vi "XY Graph Set Selected Plots.vi"(8 "Error In":errorcluster, 9 "Selected Plots":i32[](array[numeric]), 11 "XY Graph Refnum":T1) -> (0 "Error Out":errorcluster, 1 "Selected Plot Names":string[](array[string]), 2 "Caption (or Label) Text":string, 3 "XY Graph Refnum (dup)":T1)   [LabVIEW 2021, in "XY Graph Add-Ons.lvlib"]
uses:
  XY Graph Refnum.ctl
  XY Graph Add-Ons.lvlib
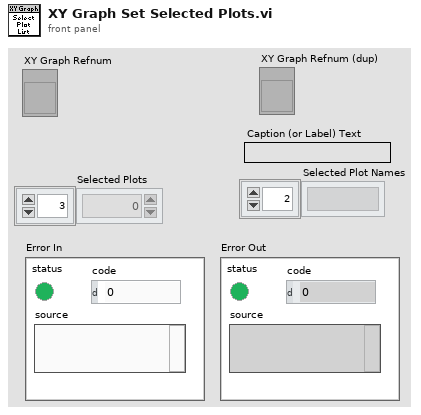
[diagram p1: front panel]
types:
  T1 = typedef "XY Graph Add-Ons.lvlib/XY Graph Refnum.ctl" = refnum<vi>
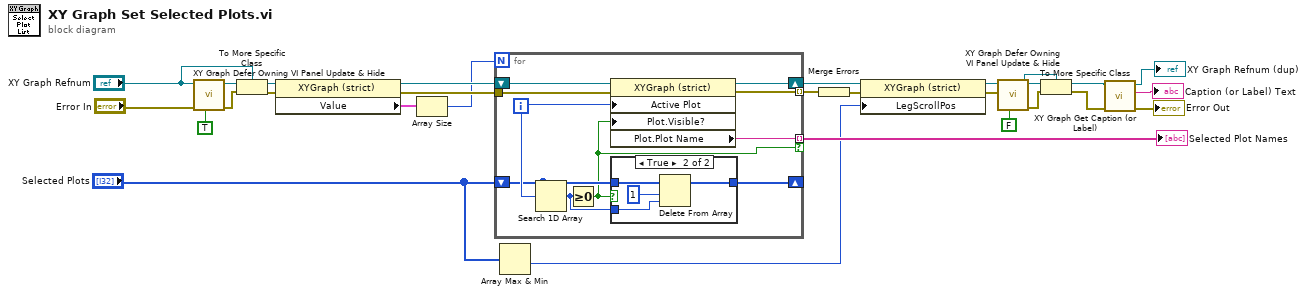
[diagram p0: block diagram]
diagram:
  n1 = call "XY Graph Defer Owning VI Panel Update & Hide.vi"("Defer Owning Panel Update"=TRUE ("Hide (F)/Show (T) Graph"), "error in (no error)"="Error In", "XY Graph Refnum in"="XY Graph Refnum") -> ("error out"=w19:errorcluster, "XY Graph Refnum out"=w21:refnum<vi>)  [unwired: 7 in]
  n2 = To More Specific Class(target class="XY Graph Refnum", reference=w21, error in=w19) -> (specific class reference=w20:T1, error out=w18:errorcluster)
  n3 = property class="XYGraph (strict)"(reference=w20, error in=w18) -> (reference out=w16:T1, error out=w22:errorcluster, "Value"=w15:cluster{"X Array":dbl[], "Y Array":dbl[]}[])
  n4 = Array Size(array=w15) -> (size(s)=w14:i32)
  n5 = for {
    N: w14 -> [_]
    shift-right: [w35] -> w4
    shift-left: w16 -> [w37]
    tunnel: w22 -> [w36]
    shift-right: [w28] -> _
    shift-left: "Selected Plots" -> [w32]
    tunnel: [w33] -> w11 mode=indexing if=w30
    tunnel: [w29] -> w13 mode=indexing
    i -> [w34]
    n6 = Search 1D Array(1D array=w32, element=w34) -> (index of element=w31:i32)  [unwired: 1 in]
    n7 = Greater Or Equal To 0?(x=w31) -> (x >= 0?=w30:bool)
    n8 = property class="XYGraph (strict)"(reference=w37, error in=w36, "Active Plot"=w34, "Plot.Visible?"=w30) -> (reference out=w35:T1, error out=w29:errorcluster, "Plot.Plot Name"=w33:string)
    n9 = case shown="True" w30 {
      tunnel: w32 -> [w38 w42]
      tunnel: [w38 w41] -> w28
      tunnel: w31 -> [_ w40]
      frame False {
      }
      frame True {
        n10 = Delete From Array(array=w42, length=1, index=w40) -> (array with subset deleted=w41:i32[])  [unwired: 1 out]
      }
    }
  }
  "Selected Plot Names" <- w11
  n11 = Array Max & Min(array="Selected Plots") -> (min value=w1:i32)  [unwired: 3 out]
  n12 = Merge Errors(w13) -> (w12:errorcluster)
  n13 = property class="XYGraph (strict)"(reference=w4, error in=w12, "LegScrollPos"=w1) -> (reference out=w3:T1, error out=w5:errorcluster)
  n14 = call "XY Graph Defer Owning VI Panel Update & Hide.vi"("Defer Owning Panel Update"=FALSE ("Hide (F)/Show (T) Graph"), "error in (no error)"=w5, "XY Graph Refnum in"=w3) -> ("error out"=w23:errorcluster, "XY Graph Refnum out"=w24:refnum<vi>)  [unwired: 7 in]
  n15 = To More Specific Class(target class=w3, reference=w24, error in=w23) -> (specific class reference=w10:T1, error out=w9:errorcluster)
  n16 = call "XY Graph Get Caption (or Label).vi"("error in (no error)"=w9, "XYGraph in"=w10) -> ("error out"=→"Error Out":errorcluster, "Caption (or Label) Text"=→"Caption (or Label) Text":string, "XYGraph out"=→"XY Graph Refnum (dup)":T1)  [unwired: 7 in]
